vi "Dashboard Main.vi"() -> ()   [LabVIEW 2014]
uses:
  <vilib>/event_ctls.llb/eventvkey.ctl
  <vilib>/Rock Robotics/WPI/Dashboard/WPI_DashboardLogging Global.vi
  <vilib>/Rock Robotics/Network Tables/SD Write Numeric Array.vi
  <vilib>/Rock Robotics/Network Tables/SD Write Number.vi
  <vilib>/Rock Robotics/Network Tables/SD Write String Array.vi
  <vilib>/Rock Robotics/Network Tables/SD Read String Array.vi
  <vilib>/Rock Robotics/Network Tables/SD Write Boolean.vi
  <vilib>/Utility/config.llb/Write Key (String).vi
  <vilib>/Utility/config.llb/Write Key (I32).vi
  <vilib>/Utility/config.llb/NI_LVConfig.lvlib
panel:
  in  "Close Dashboard":bool
  in  "TCP":refnum<k5>
  in  "Rec Mode":enum32{"Stop", "Record", "Playback"}(radio)
  in  "Vision":u16(ring) items=["Camera Off", "USB Camera SW", "USB Camera HW", "IP Camera"]
  out "Camera IP":string
  out "Image Message":string="Timeout in Camera Communications"
  in  "Dashboard Tab":T1(tab)
  in  "Camera Settings":T2={"Frame Rate"=30, "Compression"=30, "Size"=1} {"Frame Rate" scale=1.0..30.0; "Size" items=["640x480", "320x240", "160x120"]}
  out "MotorChart R":cluster{"Numeric":dbl, "Numeric":dbl}(graph)
  out "MotorChart L":T3(graph)
  out "MotorSliders R":cluster{"MotorSlide1":dbl, "MotorSlide2":dbl} {"MotorSlide2" scale=-1.0..1.0 scale format="%#_2e"; "MotorSlide1" scale=-1.0..1.0 scale format="%#_2e"}
  out "MotorSliders L":T4 {"MotorSlide4 2" scale=0.0..14.0 scale format="%#_2e"; "MotorSlide2" scale=-1.0..1.0 scale format="%#_2e"; "MotorSlide1" scale=-1.0..1.0 scale format="%#_2e"}
  out "JS1 Z":dbl(slide) scale=-1.0..1.0 scale format="%#_2e"
  out "JS1 Graph":cluster{"X":dbl, "Y":dbl}[](graph)
  out "JS1 Buttons":T5
  out "JS2 Z":dbl(slide) scale=-1.0..1.0 scale format="%#_2e"
  out "JS2 Graph":cluster{"X":dbl, "Y":dbl}[](graph)
  out "JS2 Buttons":T5
  out "Mode":T6(ring)=enum."Auto Disabled"
  in  "DB Camera Config":bool
  out "fps":dbl format="%#.1g"
  out "Mbps":dbl format="%#.1g"
  out "Mbps 2":bool
  out "Compass":dbl(knob)
  in  "DB/String 9":string
  in  "DB/String 8":string
  in  "DB/String 7":string
  in  "DB/String 6":string
  in  "DB/String 5":string
  in  "DB/String 4":string
  in  "DB/String 3":string
  in  "DB/String 2":string
  in  "DB/String 1":string
  in  "DB/String 0":string
  in  "DB/Slider 0":dbl(slide) scale=0.0..5.0
  in  "DB/Slider 1":dbl(slide) scale=0.0..5.0
  in  "DB/Slider 2":dbl(slide) scale=0.0..5.0
  in  "DB/Slider 3":dbl(slide) scale=0.0..5.0
  out "DB/LED 3":bool
  out "DB/LED 2":bool
  out "DB/LED 1":bool
  out "DB/LED 0":bool
  in  "DB/Button 3":bool
  in  "DB/Button 2":bool
  in  "DB/Button 1":bool
  in  "DB/Button 0":bool caption="New Name"
  in  "Clear Faults Joysticks":T7(ring)=enum."7 Left"
  in  "Toggle Field Centric \nJoysticks":T7(ring)=enum."3 Right"
  in  "Drive Reduction Joysticks":T7(ring)
  in  "Gyro Reset Joysticks":T7(ring)=enum."3 Left"
  in  "Toggle Field Centric\nXbox":T8(ring)=enum."Left bumper"
  in  "Gyro reset Xbox":T8(ring)=enum."Left bumper"
  in  "Drive reduction Xbox":T8(ring)=enum."Left bumper"
  in  "Clear Faults Xbox":T8(ring)=enum."Left bumper"
  in  "Rotate Joysticks":T9(ring)=enum."X right"
  in  "Translate Y Joysticks":T9(ring)=enum."Y left"
  in  "Translate X Joysticks":T9(ring)
  in  "Rotate Xbox":T10(ring)=enum."Right X"
  in  "Translate Y Xbox":T10(ring)
  in  "Translate X Xbox":T10(ring)=enum."Left Y"
  in  "Primary Mode":enum16{"Joysticks", "Xbox"}(ring)
  in  "Low elevator":T8(ring)=enum."Left bumper"
  in  "Axis for manual Control of \narm":T10(ring)
  in  "High elevator":T8(ring)=enum."Right bumper"
  in  "Claw up":T8(ring)
  in  "Claw Down":T8(ring)=enum."B"
  in  "Axis for manual Control of Claw":T10(ring)=enum."Right X"
  in  "Rotate Claw":T10(ring)=enum."Right trigger"
  in  "Open/Close claw":T8(ring)=enum."Y"
  in  "Enable Manual Claw":T8(ring)=enum."Right bumper"
  in  "Enable Manual Elevator":T8(ring)=enum."Right bumper"
  in  "Lift":T8(ring)=enum."Right bumper"
  in  "Middle Lift":T8(ring)=enum."Right bumper"
  in  "Middle Claw":T8(ring)=enum."Right bumper"
  in  "Test Slider":dbl(slide) scale=0.0..100.0 scale format="%#_3g"
  in  "On/Off":bool caption="Solenoid"
  in  "Test Name":u16(ring) items=["Select the test to run...", "Example Test", "-------------------------------", "List of tests is built in robot code.", "Replace with your own automated tests."]
  in  "Test Tree":string(tree)
  in  "Motor":cluster{"Value":dbl, "Enable":bool} {"Value" scale=-1.0..1.0 scale format="%#_3g"}
  out "Progress":T11 {"Test Progress" scale=0.0..100.0}
  in  "Rev/Fwd":cluster{"Forward":bool, "Reverse":bool}
  in  "Test Ring":u16(ring) items=["Monochrome", "Color"]
  in  "Listbox":i32(listbox)
  out "Tree":string(tree)
  in  "?":bool
  in  "Variables":string[](array[string])
  out "Camera Image":T12(plugin-control)
  out "Boolean":bool
  # "Left"
  # "Front"
  # "Right"
  # "Battery"
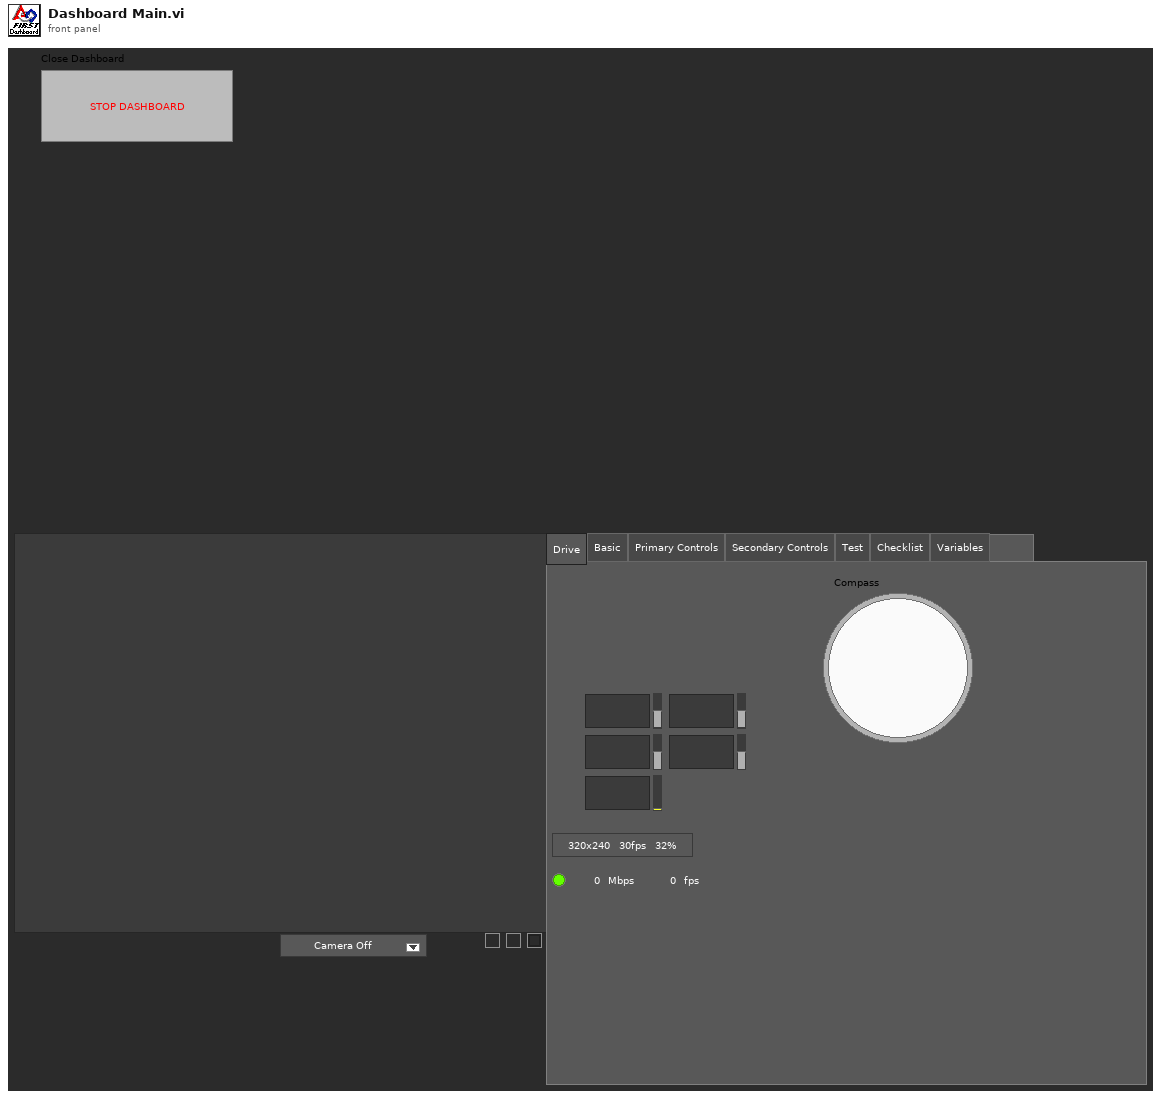
[diagram p1: front panel]
types:
  T1 = enum32{"Drive", "Basic", "Primary Controls", "Secondary Controls", "Test", "Checklist", "Variables"}
  T2 = cluster{"Frame Rate":i32, "Compression":i32, "Size":u16}
  T3 = cluster{"Numeric":dbl, "Numeric":dbl, "Battery V":dbl}
  T4 = cluster{"MotorSlide1":dbl, "MotorSlide2":dbl, "MotorSlide4 2":dbl}
  T5 = cluster{bool, bool, bool, bool, bool, bool, bool, bool, bool, bool, bool, bool}
  T6 = enum8{"Tele-Op Disabled", "Tele-Op Enabled", "Auto Disabled", "Auto Enabled", "Test Disabled", "Test Enabled", "Disconnected", "No Code", "E-Stop"}
  T7 = enum16{"Trigger Left", "2 Left", "3 Left", "4 Left", "5 Left", "6 Left", "7 Left", "8 Left", "9 Left", "10 Left", "11 Left", "Trigger Right", "2 Right", "3 Right", "4 Right", "5 Right", "6 Right", "7 Right", "8 Right", "9 Right", "10 Right", "11 Right"}
  T8 = enum16{"A", "B", "X", "Y", "Left bumper", "Right bumper", "Back", "Start", "Left Joystick down", "Right Joystick down"}
  T9 = enum16{"X left ", "Y left", "Z left", "X right", "Y right", "Z right"}
  T10 = enum16{"Left X", "Left Y", "Left trigger", "Right trigger", "Right X", "Right Y"}
  T11 = cluster{"Test Progress":u8, "Test Progress Text":string}
  T12 = typedef "IMAQ Image.ctl" = refnum<image>
  T13 = enum32{"Drive", "Basic", "Custom", "Test", "Checklist", "Variables"}
  T14 = typedef "Image Type" = u32
  T15 = enum16{"X left ", "Y left", "Z left", "X right", "Y right", "Z right"}[]
  T16 = enum16{"Trigger Left", "2 Left", "3 Left", "4 Left", "5 Left", "6 Left", "7 Left", "8 Left", "9 Left", "10 Left", "11 Left", "Trigger Right", "2 Right", "3 Right", "4 Right", "5 Right", "6 Right", "7 Right", "8 Right", "9 Right", "10 Right", "11 Right"}[]
  T17 = enum16{"Left X", "Left Y", "Left trigger", "Right trigger", "Right X", "Right Y"}[]
  T18 = enum16{"A", "B", "X", "Y", "Left bumper", "Right bumper", "Back", "Start", "Left Joystick down", "Right Joystick down"}[]
  T19 = cluster{"Error Strings":string, "Disable Counts":cluster{u16, u16}, "Rail Faults":cluster{u16, u16, u16}, "Robot IP":string, "DB Mode":u8, "Event Info":cluster{"Name":string, "Type":u8, "Number":u16, "Replay":u8}, "Camera Addr":string}
  T20 = cluster{"Storage":cluster{"Disk Free":u64, "RAM Block":u32, "RAM free":u32}, "CPU Utilization":cluster{"CPU % ISR":sgl, "CPU % Time Crit":sgl, "CPU % Timed Str":sgl, "CPU % High":sgl, "CPU % Above":sgl, "CPU % Normal":sgl, "CPU % Low":sgl}, "CAN":cluster{"% Bus Utilization":sgl, "Bus Off Cnt":u32, "TX_FIFO Full Cnt":u32, "Receive Error Cnt":u8, "Transmit Error Cnt":u8}, "HID":cluster{"HID Outputs":u32, "Rumble Low":u16, "Rumble High":u16}[]}
  T21 = cluster{"Status bits":cluster{"Test Mode":bool, "Autonomous":bool, "Enabled":bool, "Code Start":bool, "Brownout":bool, "Reserved 2":bool, "Reserved 3":bool, "E-Stop":bool}, "Code Trace":cluster{"Disabled":bool, "TeleOp":bool, "Auto":bool, "Test":bool}, "Controller Type":enum16{"unknown", "cRIO", "roboRio"}, "Code?":enum16{"unknown", "noCode", "code"}, "Battery V":dbl}
  T22 = cluster{"Control Bits":cluster{"TestMode":bool, "Autonomous":bool, "Enabled":bool, "FMS Present":bool, bool, bool, bool, "E-Stop":bool}, "Team Station ":u8, "Countdown":sgl, "Joystick Values":cluster{"Axes":dbl[], "Buttons":bool[], "POVs":i16[]}[]}
  T23 = cluster{"Axes":dbl[], "Buttons":bool[], "POVs":i16[]}[]
  T24 = cluster{"Axes":dbl[], "Buttons":bool[], "POVs":i16[]}
  T25 = cluster{"Buttons[0]":bool, "Buttons[1]":bool, "Buttons[2]":bool, "Buttons[3]":bool, "Buttons[4]":bool, "Buttons[5]":bool, "Buttons[6]":bool, "Buttons[7]":bool, "Buttons[8]":bool, "Buttons[9]":bool, "Buttons[10]":bool, "Buttons[11]":bool}
  T26 = cluster{"Camera Image":refnum<vi>, "Dashboard Tab":refnum<vi>, "Boolean":refnum<vi>, "Vision":refnum<vi>, "Rec Mode":refnum<vi>, "Test Slider":refnum<vi>, "On/Off ":refnum<vi>, "Test Ring":refnum<vi>, "Rev/Fwd":refnum<vi>, "Test Name":refnum<vi>, "Motor":refnum<vi>, "Progress":refnum<vi>, "CheckList":refnum<vi>, "Tree":refnum<vi>, "Test Tree":refnum<vi>}
  T27 = typedef "NI_LVConfig.lvlib/Config Data RefNum.ctl" = refnum<k1>
  T28 = cluster{"Operation":enum16{"Update", "Clear"}, "Color Box":u32}[]
  T29 = typedef "eventvkey.ctl" = enum16{"ASCII", "Enter", "Return", "Shift", "Ctrl", "Alt", "Cmd", "Opt", "Caps", "NumLock", "Clear", "Break", "Up", "Down", "Left", "Right", "Insert", "Delete", "Home", "End", "PageUp", "PageDown", "Escape", "Help", "Pause", "ScrollLock", "F1", "F2", "F3", "F4", "F5", "F6", "F7", "F8", "F9", "F10", "F11", "F12", "F13", "F14", "F15", "F16", "F17", "F18", "F19", "F20", "F21", "F22", "F23", "F24", "Play", "VolumeUp", "VolumeDown", "Mute", "Two Byte Char"}
  T30 = cluster{"Image Size":bool, "Image Type":bool, "Pixel Value":bool, "ROI Information":bool, "Zoom Factor":bool}
  T31 = enum8{"Enabled", "Disabled", "Disabled and Grayed Out"}
  T32 = cluster{"Operation":enum16{"Update", "Clear"}, "Color Box":u32}
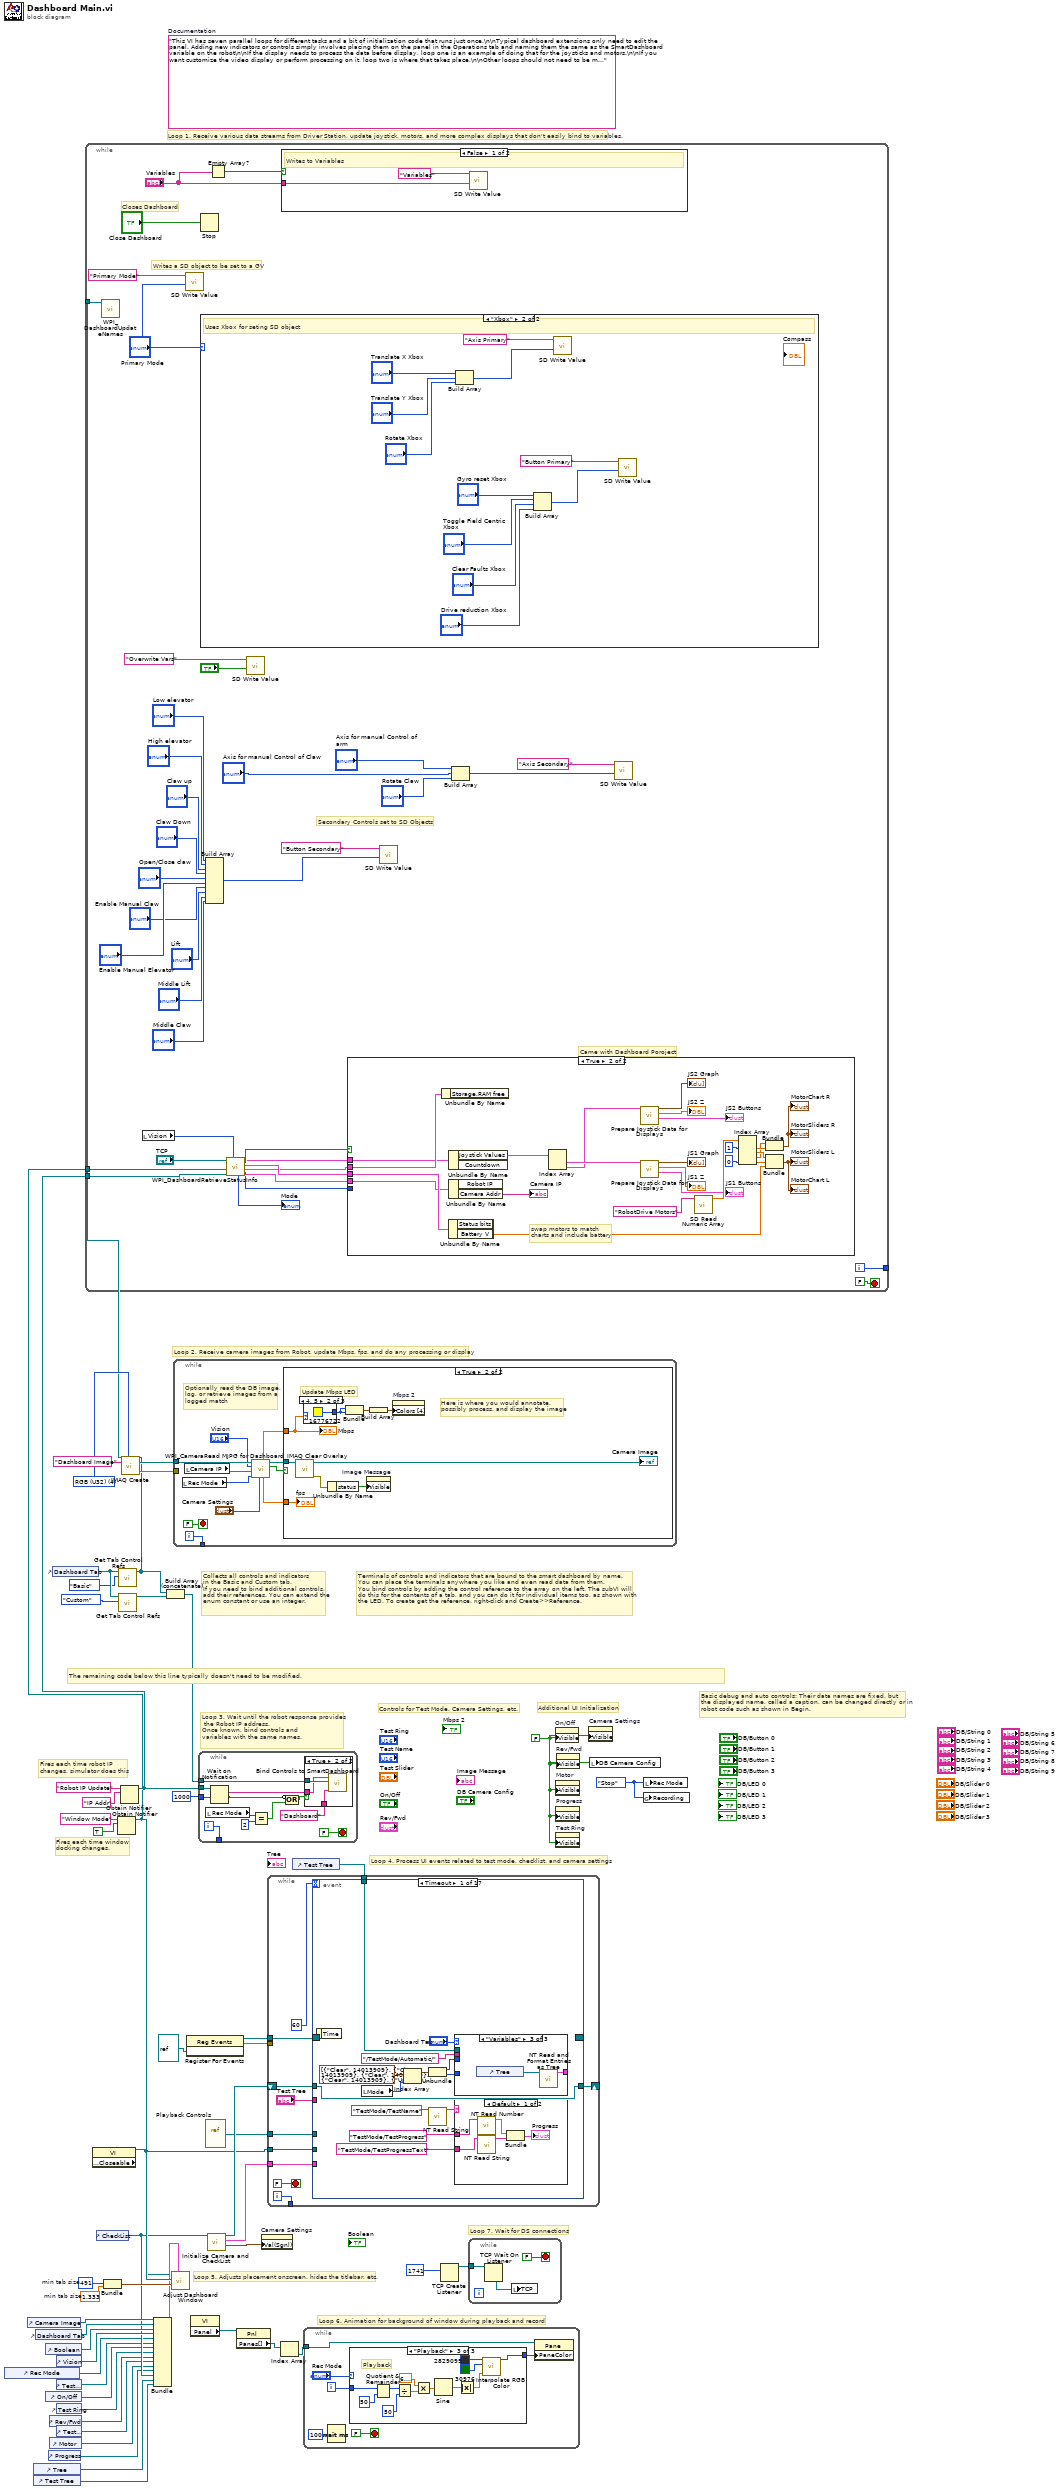
[diagram p0: block diagram]
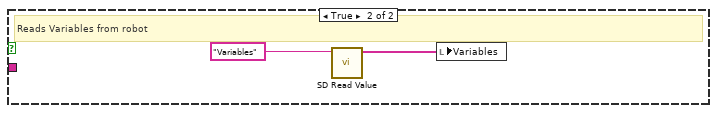
[diagram p2: hidden frame]
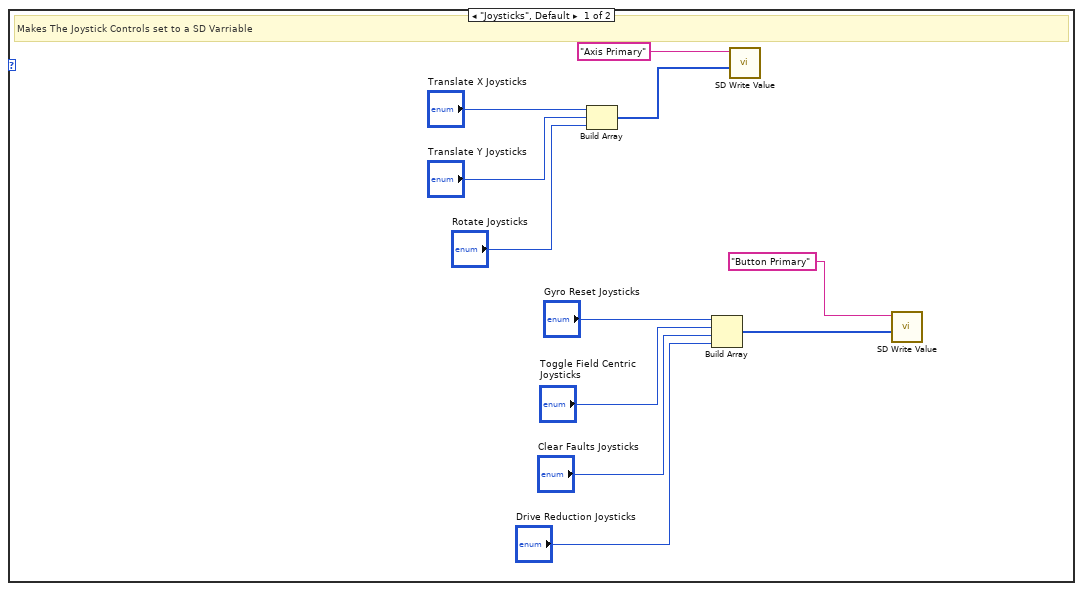
[diagram p3: hidden frame]
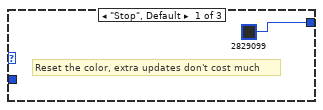
[diagram p5: hidden frame]
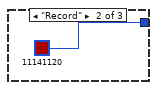
[diagram p6: hidden frame]
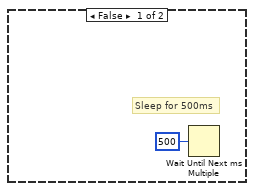
[diagram p8: hidden frame]
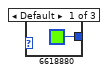
[diagram p9: hidden frame]
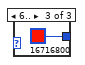
[diagram p10: hidden frame]
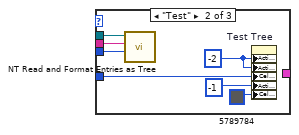
[diagram p12: hidden frame]
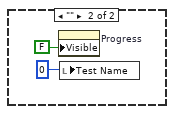
[diagram p13: hidden frame]
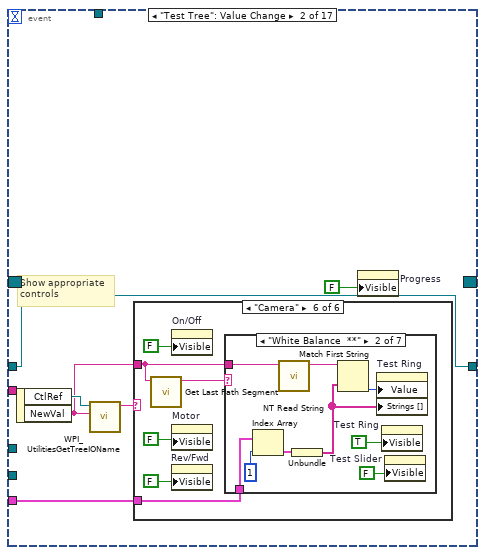
[diagram p14: hidden frame]
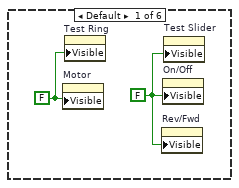
[diagram p15: hidden frame]
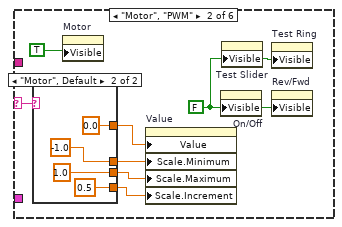
[diagram p16: hidden frame]
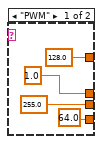
[diagram p17: hidden frame]
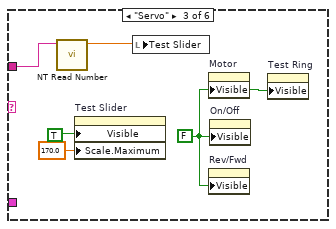
[diagram p18: hidden frame]
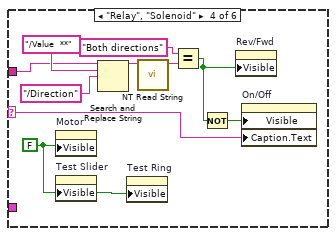
[diagram p19: hidden frame]
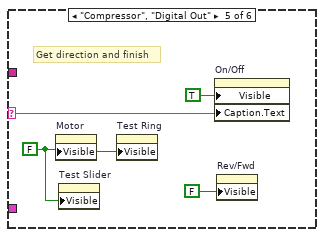
[diagram p20: hidden frame]
diagram:
  w24 = 491  # min tab size
  w23 = 1.333  # min tab size
  w32 = enum32{"Stop", "Record", "Playback"}."Stop" ("Rec Mode")
  w6 = FALSE ("Visible")
  (unwired) "This VI has seven parallel loops for different tasks and a bit of initialization code that runs just once.\n\nTypical dashboard extensions only need to edit the panel. Adding new indicators or controls simply involves placing them on the panel in the Operations tab and naming them the same as the SmartDashboard variable on the robot\n\nIf the display needs to process the data before display, loop one is an example of doing that for the joysticks and motors.\n\nIf you want customize the video display or perform processing on it, loop two is where that takes place.\n\nOther loops should not need to be modified. They are pretty standard, and document the task they perform."  # Documentation
  w52 = T14 4 items=["Grayscale (U8)", "Grayscale (I16)", "Grayscale (SGL)", "Complex (CSG)", "RGB (U32)", "HSL (U32)", "RGB (U64)"] ("Image Type")
  # "Loop 7. Wait for DS connections"
  # "Basic debug and auto controls: Their data names are fixed, but\nthe displayed name, called a caption, can be changed directly or in\nrobot code such as shown in Begin."
  # "Controls for Test Mode, Camera Settings, etc."
  # "Additional UI Initialization"
  # "Loop 6. Animation for background of window during playback and record"
  # "Fires each time robot IP\nchanges, simulator does this"
  # "Fires each time window\ndocking changes."
  # "Collects all controls and indicators\nin the Basic and Custom tab.\nIf you need to bind additional controls,\nadd their references. You can extend the\nenum constant or use an integer."
  # "The remaining code below this line typically doesn't need to be modified."
  # "Loop 4. Process UI events related to test mode, checklist, and camera settings"
  # "Terminals of controls and indicators that are bound to the smart dashboard by name.\nYou can place the terminals anywhere you like and even read data from them.\nYou bind controls by adding the control reference to the array on the left. The subVI will\ndo this for the contents of a tab, and you can do it for individual items too, as shown with\nthe LED. To create get the reference, right-click and Create>>Reference."
  # "Loop 3. Wait until the robot response provides\n the Robot IP address.\nOnce known, bind controls and\nvariables with the same names."
  # "Loop 5. Adjusts placement onscreen, hides the titlebar, etc."
  # "Loop 1. Receive various data streams from Driver Station, update joystick, motors, and more complex displays that don't easily bind to variables."
  # "Loop 2. Receive camera images from Robot, update Mbps, fps, and do any processing or display"
  n1 = control-ref of="Rec Mode"() -> (w12:refnum<vi>)
  n2 = control-ref of="Camera Image"() -> (w27:refnum<vi>)
  n3 = control-ref of="Tree"() -> (w16:refnum<vi>)
  n4 = control-ref of="Test Tree"() -> (w15:refnum<vi>)
  n5 = control-ref of="Dashboard Tab"() -> (w26:refnum<vi>)
  n6 = control-ref of="Boolean"() -> (w21:refnum<vi>)
  n7 = control-ref of="On/Off"() -> (w10:refnum<vi>)
  n8 = control-ref of="Progress"() -> (w7:refnum<vi>)
  n9 = control-ref of="Rev/Fwd"() -> (w8:refnum<vi>)
  n10 = control-ref of="Motor"() -> (w13:refnum<vi>)
  n11 = control-ref of="Dashboard Tab"() -> (w30:refnum<vi>)
  n12 = control-ref of="Test Slider"() -> (w11:refnum<vi>)
  n13 = control-ref of="Vision"() -> (w25:refnum<vi>)
  n14 = control-ref of="Test Ring"() -> (w9:refnum<vi>)
  n15 = control-ref of="Test Name"() -> (w14:refnum<vi>)
  n16 = property class="VI" props=["Front Panel.Closeable"]() -> (reference out=w31:refnum<vi>)  [unwired: 2 in, 2 out]
  n17 = control-ref of="CheckList"() -> (w17:refnum<vi>)
  n18 = Bundle("min tab size"=w24, "min tab size"=w23) -> (w22:cluster{"min tab size":i32, "min tab size":dbl})  [unwired: 1 in]
  n19 = Obtain Notifier(name (unnamed)="Window Mode", notification data type=TRUE) -> (notifier out=w3:refnum<notifier>)  [unwired: 2 in, 2 out]
  n20 = call <vilib>:"Get Tab Control Refs.vi"("Page Index"=T13."Basic" ("Dashboard Tab"), "TabControl in"=w30) -> ("ControlsOnPage"=w4:refnum<vi>[])  [unwired: 9 in]
  n21 = call <vilib>:"Get Tab Control Refs.vi"("Page Index"=T13."Custom" ("Dashboard Tab"), "TabControl in"=w30) -> ("ControlsOnPage"=w29:refnum<vi>[])  [unwired: 9 in]
  n22 = Obtain Notifier(name (unnamed)="Robot IP Update", notification data type="IP Addr" ("name (unnamed)")) -> (notifier out=w5:refnum<notifier>)  [unwired: 2 in, 2 out]
  n23 = while {
    tunnel: [w88] -> _
    tunnel: w5 -> [w82]
    tunnel: w4 -> [w81]
    tunnel: w3 -> [w77]
    i -> [w88]
    stop <- FALSE stop-if-true
    # "Closes Dashboard"
    # "Came with Dashboard Poroject"
    # "Writes a SD object to be set to a GV"
    # "Secondary Controls set to SD Objects"
    n24 = call <vilib>:"WPI_DashboardUpdateNames.vi"("Controls on Tab"=w81) -> ()  [unwired: 11 in]
    n25 = local read "Vision"() -> (w79:u16)
    n26 = call-poly <vilib>:"SD Write Value.vi"("Numeric"="Primary Mode", "Name"="Primary Mode") -> ()  [unwired: 8 in, 2 out]
    n27 = Stop(stop? (T)="Close Dashboard") -> ()
    n28 = case shown="\"Xbox\"" "Primary Mode" {
      frame "Joysticks", Default {
        # "Makes The Joystick Controls set to a SD Varriable"
        n29 = Build Array("Translate X Joysticks", "Translate Y Joysticks", "Rotate Joysticks") -> (w104:T15)
        n30 = Build Array("Gyro Reset Joysticks", "Toggle Field Centric \nJoysticks", "Clear Faults Joysticks", "Drive Reduction Joysticks") -> (w97:T16)
        n31 = call-poly <vilib>:"SD Write Value.vi"("Numeric Array"=w104, "Name"="Axis Primary") -> ()  [unwired: 8 in, 2 out]
        n32 = call-poly <vilib>:"SD Write Value.vi"("Numeric Array"=w97, "Name"="Button Primary") -> ()  [unwired: 8 in, 2 out]
      }
      frame "Xbox" {
        # "Uses Xbox for seting SD object"
        n33 = Build Array("Translate X Xbox", "Translate Y Xbox", "Rotate Xbox") -> (w112:T17)
        n34 = Build Array("Gyro reset Xbox", "Toggle Field Centric\nXbox", "Clear Faults Xbox", "Drive reduction Xbox") -> (w115:T18)
        n35 = call-poly <vilib>:"SD Write Value.vi"("Numeric Array"=w112, "Name"="Axis Primary") -> ()  [unwired: 8 in, 2 out]
        n36 = call-poly <vilib>:"SD Write Value.vi"("Numeric Array"=w115, "Name"="Button Primary") -> ()  [unwired: 8 in, 2 out]
      }
    }
    n37 = Build Array("Low elevator", "High elevator", "Claw up", "Claw Down", "Open/Close claw", "Enable Manual Elevator", "Enable Manual Claw", "Lift", "Middle Lift", "Middle Claw") -> (w75:T18)
    n38 = Empty Array?(array="Variables") -> (empty?=w59:bool)
    n39 = call <vilib>:"WPI_DashboardRetrieveStatusInfo.vi"("Vision"=w79, "Binding Refnum"=w82, "Window Mode Notifier"=w77, "TCP Cnx"="TCP") -> ("Power and Errors"=w83:T19, "Robot Metrics"=w86:T20, "Status Info"=w87:T21, "Control Info"=w84:T22, "Robot Mode"=w80:T6, "Process?"=w85:bool)  [unwired: 2 in]
    "Mode" <- w80
    n40 = call-poly <vilib>:"SD Write Value.vi"("Boolean"="?", "Name"="Overwrite Vars") -> ()  [unwired: 8 in, 2 out]
    n41 = case shown="False" w59 {
      tunnel: "Variables" -> [w90 _]
      frame False {
        # "Writes to Variables"
        n42 = call-poly <vilib>:"SD Write Value.vi"("String Array"=w90, "Name"="Variables") -> ()  [unwired: 8 in, 2 out]
      }
      frame True {
        # "Reads Variables from robot"
        n43 = call-poly <vilib>:"SD Read Value.vi"("Name"="Variables") -> ("String Array"=w92:string[])  [unwired: 9 in, 1 out]
        n44 = local write "Variables"(w92) -> ()
      }
    }
    n45 = case shown="True" w85 {
      tunnel: w87 -> [_ w140]
      tunnel: w86 -> [_ w139]
      tunnel: w84 -> [_ w138]
      tunnel: w83 -> [_ w137]
      tunnel: w80 -> [_ _]
      frame False {
      }
      frame True {
        # "swap motors to match\ncharts and include battery"
        n46 = Unbundle By Name(w139) -> ()  [unwired: 1 out]
        n47 = Unbundle By Name(w140) -> ("Battery V"=w126:dbl)  [unwired: 1 out]
        n48 = Unbundle By Name(w138) -> ("Joystick Values"=w125:T23)  [unwired: 1 out]
        n49 = Unbundle By Name(w137) -> ("Camera Addr"=→"Camera IP":string)  [unwired: 1 out]
        n50 = Index Array(array=w125) -> (element #1=w124:T24, element #2=w119:T24)  [unwired: 2 in]
        n51 = call "Prepare Joystick Data for Displays.vi"("Joystick Values"=w119) -> ("Buttons"=→"JS2 Buttons":T25, "Z Axis"=→"JS2 Z":dbl, "Cartesian Data"=→"JS2 Graph":cluster{"X axis":dbl, "X axis":dbl}[])  [unwired: 8 in]
        n52 = call "Prepare Joystick Data for Displays.vi"("Joystick Values"=w124) -> ("Buttons"=→"JS1 Buttons":T25, "Z Axis"=→"JS1 Z":dbl, "Cartesian Data"=→"JS1 Graph":cluster{"X axis":dbl, "X axis":dbl}[])  [unwired: 8 in]
        n53 = call <vilib>:"SD Read Numeric Array.vi"("Name"="RobotDrive Motors") -> ("Numeric Array"=w128:dbl[])  [unwired: 8 in, 2 out]
        n54 = Index Array(array=w128, index #1=1, index #4=0) -> (element #1=w132:dbl, element #2=w133:dbl, element #3=w131:dbl, element #4=w136:dbl)  [unwired: 2 in]
        n55 = Bundle("Numeric"=w131, "Numeric"=w132) -> (→"MotorChart R" →"MotorSliders R":cluster{"Numeric":dbl, "Numeric":dbl})  [unwired: 1 in]
        n56 = Bundle("Numeric"=w133, "Numeric"=w136, "Battery V"=w126) -> (→"MotorChart L" →"MotorSliders L":T3)  [unwired: 1 in]
      }
    }
    n57 = call-poly <vilib>:"SD Write Value.vi"("Numeric Array"=w75, "Name"="Button Secondary") -> ()  [unwired: 8 in, 2 out]
    n58 = Build Array("Axis for manual Control of \narm", "Axis for manual Control of Claw", "Rotate Claw") -> (w57:T17)
    n59 = call-poly <vilib>:"SD Write Value.vi"("Numeric Array"=w57, "Name"="Axis Secondary") -> ()  [unwired: 8 in, 2 out]
  }
  n60 = call "IMAQ Create"("Image Name"="Dashboard Image", "Image Type"=w52) -> ("New Image"=w50:T12, "error out"=w49:errorcluster)  [unwired: 2 in, 1 out]
  n61 = Bundle("Camera Image"=w27, "Dashboard Tab"=w26, "Boolean"=w21, "Vision"=w25, "Rec Mode"=w12, "Test Slider"=w11, "On/Off"=w10, "Test Ring"=w9, "Rev/Fwd"=w8, "Test Name"=w14, "Motor"=w13, "Progress"=w7, "CheckList"=w17, "Tree"=w16, "Test Tree"=w15) -> (w18:T26)  [unwired: 1 in]
  n62 = Build Array (concatenate)(w4, w29) -> (w28:refnum<vi>[])
  n63 = call "Adjust Dashboard Window.vi"("Sizing Refnums"=w18, "Size Constraints"=w22, "VI"=w31, "Notifier in"=w3) -> ()  [unwired: 8 in]
  n64 = while {
    tunnel: w50 -> [w149]
    tunnel: w49 -> [_]
    tunnel: [w150] -> _
    i -> [w150]
    stop <- FALSE stop-if-true
    # "Optionally read the DB image,\nlog, or retrieve images from a\nlogged match"
    n65 = local read "Rec Mode"() -> (w143:enum32{"Stop", "Record", "Playback"})
    n66 = local read "Camera IP"() -> (w141:string)
    n67 = call <vilib>:"WPI_CameraRead MJPG for Dashboard.vi"("Camera Settings"="Camera Settings", "Rec Mode"=w143, "Camera IP"=w141, "Camera Mode"="Vision", "Refnum in"=w149) -> ("Active"=w147:bool, "Refnum out"=w148:T12, "FPS"=w146:dbl, "Bandwidth (Mbps)"=w145:dbl)  [unwired: 3 in]
    n68 = case shown="True" w147 {
      tunnel: w148 -> [_ w156]
      tunnel: w145 -> [_ w155]
      tunnel: w146 -> [_ w153]
      frame False {
        # "Sleep for 500ms"
        n69 = Wait Until Next ms Multiple(millisecond multiple=u32 500) -> ()  [unwired: 1 out]
      }
      frame True {
        # "Here is where you would annotate,\npossibly process, and display the image"
        # "Update Mbps LED"
        n70 = call "IMAQ Clear Overlay"("Image"=w156) -> ("error out"=w160:errorcluster, "Image Out"=→"Camera Image":T12)  [unwired: 2 in, 7 out]
        n71 = case shown="4, 5" w155 {
          tunnel: [u32 6618880 ("Color Box") u32 16776722 ("Color Box") u32 16716800 ("Color Box")] -> w157
          frame Default {
          }
          frame 4, 5 {
          }
          frame 6.. {
          }
        }
        n72 = Unbundle By Name(w160) -> ("status"=w161:bool)
        n73 = Bundle("Color Box"=w157, "Color Box"=w157) -> (w159:cluster{"Color Box":u32, "Color Box":u32})  [unwired: 1 out]
        n74 = property on="Image Message" class="Str"("Visible"=w161) -> ()  [unwired: 2 in, 2 out]
        n75 = Build Array(w159) -> (w158:cluster{"Color Box":u32, "Color Box":u32}[])
        n76 = property on="Mbps 2" class="Bool (strict)"("Colors [4]"=w158) -> ()  [unwired: 2 in, 2 out]
        "Mbps" <- w155
        "fps" <- w153
      }
    }
  }
  n77 = register-events(refnum<vi> refnum) -> (reference out=w36:refnum<event-registration>, error out=w35:errorcluster)  [unwired: 2 in]
  n78 = property class="VI"() -> ("Panel"=w39:refnum<vi>)  [unwired: 2 in, 2 out]
  n79 = while {
    tunnel: w28 -> [w176]
    tunnel: w5 -> [w174]
    tunnel: [w172] -> _
    tunnel: u32 1000 ("milliseconds to wait") -> [w171]
    i -> [w172]
    stop <- FALSE stop-if-true
    n80 = local read "Rec Mode"() -> (w167:enum32{"Stop", "Record", "Playback"})
    n81 = Wait on Notification(notifier=w174, timeout in ms (-1)=w171) -> (notification=w173:string, timed out?=w169:bool)  [unwired: 2 in, 2 out]
    n82 = Equal?(x=w167, y=u16 2 ("Rec Mode")) -> (x = y?=w168:bool)
    n83 = Compound Arithmetic op=OR(invert w169, w168) -> (w170:bool)
    n84 = case shown="True" w170 {
      tunnel: w176 -> [_ w179]
      tunnel: w173 -> [_ w178]
      tunnel: "Dashboard" -> [_ w177]
      frame False {
      }
      frame True {
        n85 = call <vilib>:"Bind Controls to SmartDashboard.vi"("Client Name"=w177, "Bound Control Refs"=w179, "Server IP Address"=w178) -> ()  [unwired: 9 in]
      }
    }
  }
  n86 = vi-ref "Playback Controls.vi"() -> (w37:refnum<vi>)
  n87 = call "Initialize Camera and CheckList.vi"("ListBox in"=w17) -> ("Cluster"=w43:cluster{"value":i32, "value":i32, "index":i32}, "Array"=w44:cluster{string[]}[], "File Refnum"=w42:T27)  [unwired: 8 in]
  n88 = property class="Pnl"(reference=w39) -> ("Panes[]"=w40:refnum<vi>[])  [unwired: 1 in, 2 out]
  n89 = property on="Camera Settings" class="Clust (strict)"("Val(Sgnl)"=w43) -> ()  [unwired: 2 in, 2 out]
  n90 = Index Array(array=w40) -> (element=w38:refnum<vi>)  [unwired: 1 in]
  n91 = control-ref of="Test Tree"() -> (w41:refnum<vi>)
  n92 = while {
    tunnel: w44 -> [w187]
    shift-right: [w186] -> _
    shift-left: w42 -> [w185]
    tunnel: [w184] -> _
    tunnel: w41 -> [w183]
    tunnel: w37 -> [w182]
    tunnel: w36 -> [w181]
    tunnel: w35 -> [_]
    tunnel: w31 -> [w180]
    i -> [w184]
    stop <- FALSE stop-if-true
    n93 = event shown="[0] Timeout" {
      selector: w181 -> [_ _ _ _ _ _ _ _ _ _ _ _ _ _ _ _ _]
      dyn-events: [_ _ _ _ _ _ _ _ _ _ _ _ _ w425 _ _ _] -> _
      timeout: u32 60 ("milliseconds to wait") -> [_ _ _ _ _ _ _ _ _ _ _ _ _ _ _ _ _]
      tunnel: w183 -> [w199 _ _ _ _ _ _ _ _ _ _ _ _ _ _ _ _]
      tunnel: "Test Tree" -> [_ _ _ _ _ _ _ _ w394 w402 w404 w408 w416 _ _ _ _]
      tunnel: w187 -> [_ w221 _ _ _ _ w358 w388 _ _ _ _ _ _ _ _ _]
      tunnel: [w195 w220 w319 w324 w332 w344 w357 w381 w393 w400 w403 w407 w415 w427 w441 w442 w452] -> w186
      tunnel: w185 -> [w195 w220 w319 w324 w332 w344 w356 w381 w393 w400 w403 w407 w415 w427 w441 w442 w452]
      tunnel: w182 -> [_ _ _ _ _ _ _ _ _ _ _ _ _ w428 _ w445 _]
      tunnel: w180 -> [_ _ _ _ _ _ _ _ _ _ _ _ _ w423 _ _ _]
      event Timeout {
        n94 = event-data() -> ()  [unwired: 1 in, 1 out]
        n95 = local read "Mode"() -> (w198:T6)
        n96 = Index Array(array=T28 [{"Operation"=enum."Clear", "Color Box"=14013909}, {"Operation"=enum."Clear", "Color Box"=14013909}, {"Operation"=enum."Clear", "Color Box"=14013909}, {"Operation"=enum."Clear", "Color Box"=14013909}, {"Operation"=enum."Update", "Color Box"=14013909}, {"Operation"=enum."Update", "Color Box"=16777215}, {"Operation"=enum."Clear", "Color Box"=14013909}, {"Operation"=enum."Clear", "Color Box"=14013909}, {"Operation"=enum."Clear", "Color Box"=14013909}], index=w198) -> (element=w193:T32)
        n97 = Unbundle(w193) -> ("Operation"=w192:enum16{"Update", "Clear"}, "Color Box"=w191:u32)
        n98 = call <vilib>:"NT Read String.vi"("Name"="TestMode/TestName") -> ("String"=w202:string)  [unwired: 9 in, 1 out]
        n99 = case shown="\"Variables\"" "Dashboard Tab" {
          tunnel: w199 -> [_ w210 _]
          tunnel: "/TestMode/Automatic/" ("Name Pattern") -> [_ w209 _]
          tunnel: w192 -> [_ w208 _]
          tunnel: [_ _ w212] -> _
          tunnel: w191 -> [_ w204 _]
          frame "Primary Controls", Default {
          }
          frame "Test" {
            w207 = -2 ("Active Item:Row Number")
            n100 = call <vilib>:"NT Read and Format Entries as Tree.vi"("Operation"=w208, "Name Pattern"=w209, "Tree Refnum"=w210) -> ()  [unwired: 7 in, 2 out]
            n101 = property on="Test Tree" class="Tree (strict)"("Active Item Row Number"=w207, "ActiveColNum"=w207, "CellBG"=w204, "Active Item Row Number"=-1 ("Active Item:Row Number"), "CellBG"=u32 5789784 ("Color Box")) -> ()  [unwired: 2 in, 2 out]
          }
          frame "Variables" {
            n102 = control-ref of="Tree"() -> (w211:refnum<vi>)
            n103 = call <vilib>:"NT Read and Format Entries as Tree.vi"("Tree Refnum"=w211) -> ("Formatted Strings"=w212:cluster{"Name":string, "Value":string}[])  [unwired: 9 in, 1 out]
          }
        }
        n104 = case shown="Default" w202 {
          tunnel: "TestMode/TestProgress" ("Name") -> [w214 _]
          tunnel: "TestMode/TestProgressText" ("Name") -> [w213 _]
          frame Default {
            n105 = call <vilib>:"NT Read Number.vi"("Name"=w214) -> ("Numeric"=w215:dbl)  [unwired: 9 in, 1 out]
            n106 = call <vilib>:"NT Read String.vi"("Name"=w213) -> ("String"=w216:string)  [unwired: 9 in, 1 out]
            n107 = Bundle("Numeric"=w215, "String"=w216) -> (→"Progress":cluster{"Numeric":dbl, "String":string})  [unwired: 1 in]
          }
          frame "" {
            n108 = property on="Progress" class="Clust (strict)"("Visible"=FALSE) -> ()  [unwired: 2 in, 2 out]
            n109 = local write "Test Name"(u16 0) -> ()
          }
        }
      }
      event "Test Tree": Value Change {
        # "Show appropriate\ncontrols"
        n110 = event-data() -> ("CtlRef"=w224:refnum<vi>, "NewVal"=w222:string)  [unwired: 1 in]
        n111 = call <vilib>:"WPI_UtilitiesGetTreeIOName.vi"("NewVal"=w222, "TreeControl in"=w224) -> ("I/O Name"=w225:string)  [unwired: 9 in]
        n112 = case shown="\"Camera\"" w225 {
          selector: w225 -> [_ w232 _ w250 w259 _]
          tunnel: w222 -> [_ _ w247 w249 _ w266]
          tunnel: w221 -> [_ _ _ _ _ w265]
          frame Default {
            w227 = FALSE ("Visible")
            w226 = FALSE ("Visible")
            n113 = property on="Motor" class="Clust (strict)"("Visible"=w226) -> ()  [unwired: 2 in, 2 out]
            n114 = property on="Test Ring" class="Ring (strict)"("Visible"=w226) -> ()  [unwired: 2 in, 2 out]
            n115 = property on="Rev/Fwd" class="Clust (strict)"("Visible"=w227) -> ()  [unwired: 2 in, 2 out]
            n116 = property on="On/Off" class="Bool (strict)"("Visible"=w227) -> ()  [unwired: 2 in, 2 out]
            n117 = property on="Test Slider" class="Slide (strict)"("Visible"=w227) -> ()  [unwired: 2 in, 2 out]
          }
          frame "Motor", "PWM" {
            w233 = FALSE ("Visible")
            n118 = case shown="\"Motor\", Default" w232 {
              tunnel: [1.0 ("Value") -1.0 ("Value")] -> w231
              tunnel: [255.0 ("Value") 1.0 ("Value")] -> w230
              tunnel: [128.0 ("Value") 0.0 ("Value")] -> w229
              tunnel: [64.0 ("Value") 0.5 ("Value")] -> w228
              frame "PWM" {
              }
              frame "Motor", Default {
              }
            }
            n119 = property on="Motor" class="Clust (strict)"("Visible"=TRUE) -> ()  [unwired: 2 in, 2 out]
            n120 = property on="Value" class="Slide (strict)"("Value"=w229, "Scale.Minimum"=w231, "Scale.Maximum"=w230, "Scale.Increment"=w228) -> ()  [unwired: 2 in, 2 out]
            n121 = property on="On/Off" class="Bool (strict)"("Visible"=w233) -> ()  [unwired: 2 in, 2 out]
            n122 = property on="Test Slider" class="Slide (strict)"("Visible"=w233) -> ()  [unwired: 2 in, 2 out]
            n123 = property on="Test Ring" class="Ring (strict)"("Visible"=w233) -> ()  [unwired: 2 in, 2 out]
            n124 = property on="Rev/Fwd" class="Clust (strict)"("Visible"=w233) -> ()  [unwired: 2 in, 2 out]
          }
          frame "Servo" {
            w245 = FALSE ("Visible")
            n125 = call <vilib>:"NT Read Number.vi"("Name"=w247) -> ("Numeric"=w246:dbl)  [unwired: 9 in, 1 out]
            n126 = property on="Test Slider" class="Slide (strict)"("Visible"=TRUE, "Scale.Maximum"=170.0 ("Scale.Range:Maximum")) -> ()  [unwired: 2 in, 2 out]
            n127 = local write "Test Slider"(w246) -> ()
            n128 = property on="Motor" class="Clust (strict)"("Visible"=w245) -> ()  [unwired: 2 in, 2 out]
            n129 = property on="Rev/Fwd" class="Clust (strict)"("Visible"=w245) -> ()  [unwired: 2 in, 2 out]
            n130 = property on="On/Off" class="Bool (strict)"("Visible"=w245) -> ()  [unwired: 2 in, 2 out]
            n131 = property on="Test Ring" class="Ring (strict)"("Visible"=w245) -> ()  [unwired: 2 in, 2 out]
          }
          frame "Relay", "Solenoid" {
            w248 = FALSE ("Visible")
            n132 = property on="Motor" class="Clust (strict)"("Visible"=w248) -> ()  [unwired: 2 in, 2 out]
            n133 = property on="Test Slider" class="Slide (strict)"("Visible"=w248) -> ()  [unwired: 2 in, 2 out]
            n134 = Search and Replace String(input string=w249, search string="/Value  **", replace string="/Direction") -> (result string=w255:string)  [unwired: 5 in, 3 out]
            n135 = property on="Test Ring" class="Ring (strict)"("Visible"=w248) -> ()  [unwired: 2 in, 2 out]
            n136 = call <vilib>:"NT Read String.vi"("Name"=w255) -> ("String"=w253:string)  [unwired: 9 in, 1 out]
            n137 = Equal?(x="Both directions", y=w253) -> (x = y?=w251:bool)
            n138 = Not(x=w251) -> (.not. x?=w252:bool)
            n139 = property on="Rev/Fwd" class="Clust (strict)"("Visible"=w251) -> ()  [unwired: 2 in, 2 out]
            n140 = property on="On/Off" class="Bool (strict)"("Visible"=w252, "Caption.Text"=w250) -> ()  [unwired: 2 in, 2 out]
          }
          frame "Compressor", "Digital Out" {
            w258 = FALSE ("Visible")
            # "Get direction and finish"
            n141 = property on="Motor" class="Clust (strict)"("Visible"=w258) -> ()  [unwired: 2 in, 2 out]
            n142 = property on="Test Slider" class="Slide (strict)"("Visible"=w258) -> ()  [unwired: 2 in, 2 out]
            n143 = property on="Test Ring" class="Ring (strict)"("Visible"=w258) -> ()  [unwired: 2 in, 2 out]
            n144 = property on="On/Off" class="Bool (strict)"("Visible"=TRUE, "Caption.Text"=w259) -> ()  [unwired: 2 in, 2 out]
            n145 = property on="Rev/Fwd" class="Clust (strict)"("Visible"=FALSE) -> ()  [unwired: 2 in, 2 out]
          }
          frame "Camera" {
            n146 = call <vilib>:"Get Last Path Segment.vi"("String in"=w266) -> ("String out"=w267:string)  [unwired: 10 in]
            n147 = property on="On/Off" class="Bool (strict)"("Visible"=FALSE) -> ()  [unwired: 2 in, 2 out]
            n148 = property on="Motor" class="Clust (strict)"("Visible"=FALSE) -> ()  [unwired: 2 in, 2 out]
            n149 = property on="Rev/Fwd" class="Clust (strict)"("Visible"=FALSE) -> ()  [unwired: 2 in, 2 out]
            n150 = case shown="\"White Balance  **\"" w267 {
              tunnel: w266 -> [w273 w282 w291 w300 w309 _ w315]
              tunnel: w265 -> [w271 w279 w288 w297 w306 _ _]
              frame "Size  **" {
                n151 = Index Array(array=w271) -> (element=w270:cluster{string[]})  [unwired: 1 in]
                n152 = call <vilib>:"NT Read String.vi"("Name"=w273) -> ("String"=w272:string)  [unwired: 9 in, 1 out]
                n153 = Unbundle(w270) -> (w268:string[])
                n154 = Match First String(2:w268, 3:w272) -> (0:w269:i32)  [unwired: 1 out]
                n155 = property on="Test Ring" class="Ring (strict)"("Value"=w269, "Strings []"=w268) -> ()  [unwired: 2 in, 2 out]
                n156 = property on="Test Ring" class="Ring (strict)"("Visible"=TRUE) -> ()  [unwired: 2 in, 2 out]
                n157 = property on="Test Slider" class="Slide (strict)"("Visible"=FALSE) -> ()  [unwired: 2 in, 2 out]
              }
              frame "White Balance  **" {
                n158 = Index Array(array=w279, index=1) -> (element=w280:cluster{string[]})
                n159 = call <vilib>:"NT Read String.vi"("Name"=w282) -> ("String"=w281:string)  [unwired: 9 in, 1 out]
                n160 = Unbundle(w280) -> (w277:string[])
                n161 = Match First String(2:w277, 3:w281) -> (0:w276:i32)  [unwired: 1 out]
                n162 = property on="Test Ring" class="Ring (strict)"("Value"=w276, "Strings []"=w277) -> ()  [unwired: 2 in, 2 out]
                n163 = property on="Test Ring" class="Ring (strict)"("Visible"=TRUE) -> ()  [unwired: 2 in, 2 out]
                n164 = property on="Test Slider" class="Slide (strict)"("Visible"=FALSE) -> ()  [unwired: 2 in, 2 out]
              }
              frame "Exposure  **" {
                n165 = Index Array(array=w288, index=2) -> (element=w289:cluster{string[]})
                n166 = call <vilib>:"NT Read String.vi"("Name"=w291) -> ("String"=w290:string)  [unwired: 9 in, 1 out]
                n167 = Unbundle(w289) -> (w285:string[])
                n168 = Match First String(2:w285, 3:w290) -> (0:w286:i32)  [unwired: 1 out]
                n169 = property on="Test Ring" class="Ring (strict)"("Value"=w286, "Strings []"=w285) -> ()  [unwired: 2 in, 2 out]
                n170 = property on="Test Ring" class="Ring (strict)"("Visible"=TRUE) -> ()  [unwired: 2 in, 2 out]
                n171 = property on="Test Slider" class="Slide (strict)"("Visible"=FALSE) -> ()  [unwired: 2 in, 2 out]
              }
              frame "Exposure Priority  **" {
                n172 = Index Array(array=w297, index=3) -> (element=w298:cluster{string[]})
                n173 = call <vilib>:"NT Read String.vi"("Name"=w300) -> ("String"=w299:string)  [unwired: 9 in, 1 out]
                n174 = Unbundle(w298) -> (w294:string[])
                n175 = Match First String(2:w294, 3:w299) -> (0:w295:i32)  [unwired: 1 out]
                n176 = property on="Test Ring" class="Ring (strict)"("Value"=w295, "Strings []"=w294) -> ()  [unwired: 2 in, 2 out]
                n177 = property on="Test Ring" class="Ring (strict)"("Visible"=TRUE) -> ()  [unwired: 2 in, 2 out]
                n178 = property on="Test Slider" class="Slide (strict)"("Visible"=FALSE) -> ()  [unwired: 2 in, 2 out]
              }
              frame "Color Enable  **" {
                n179 = Index Array(array=w306, index=4) -> (element=w307:cluster{string[]})
                n180 = call <vilib>:"NT Read String.vi"("Name"=w309) -> ("String"=w308:string)  [unwired: 9 in, 1 out]
                n181 = Unbundle(w307) -> (w303:string[])
                n182 = Match First String(2:w303, 3:w308) -> (0:w304:i32)  [unwired: 1 out]
                n183 = property on="Test Ring" class="Ring (strict)"("Value"=w304, "Strings []"=w303) -> ()  [unwired: 2 in, 2 out]
                n184 = property on="Test Ring" class="Ring (strict)"("Visible"=TRUE) -> ()  [unwired: 2 in, 2 out]
                n185 = property on="Test Slider" class="Slide (strict)"("Visible"=FALSE) -> ()  [unwired: 2 in, 2 out]
              }
              frame Default {
                n186 = property on="Test Ring" class="Ring (strict)"("Visible"=FALSE) -> ()  [unwired: 2 in, 2 out]
                n187 = property on="Test Slider" class="Slide (strict)"("Visible"=FALSE) -> ()  [unwired: 2 in, 2 out]
              }
              frame "Brightness  **", "Color Level  **", "Compression  **", "FPS  **", "Sharpness  **" {
                n188 = call <vilib>:"NT Read Number.vi"("Name"=w315) -> ("Numeric"=w314:dbl)  [unwired: 9 in, 1 out]
                n189 = local write "Test Slider"(w314) -> ()
                n190 = property on="Test Slider" class="Slide (strict)"("Visible"=TRUE, "Scale.Maximum"=100.0 ("Scale.Range:Maximum")) -> ()  [unwired: 2 in, 2 out]
                n191 = property on="Test Ring" class="Ring (strict)"("Visible"=FALSE) -> ()  [unwired: 2 in, 2 out]
              }
            }
          }
        }
        n192 = property on="Progress" class="Clust (strict)"("Visible"=FALSE) -> ()  [unwired: 2 in, 2 out]
      }
      event "Test Name": Mouse Enter {
        # "Populate the ring with the list of tests"
        n193 = event-data() -> ()  [unwired: 1 in, 1 out]
        n194 = call <vilib>:"NT Read String Array.vi"("Name"="TestMode/TestList") -> ("String Array"=w323:string[])  [unwired: 9 in, 1 out]
        n195 = Build Array (concatenate)("Select the test to run...", w323) -> (w322:string[])
        n196 = property on="Test Name" class="Ring (strict)"("Strings []"=w322) -> ()  [unwired: 2 in, 2 out]
      }
      event "Test Name": Value Change {
        w325 = FALSE ("Visible")
        # "Tell the robot the test name to run"
        n197 = event-data() -> ("NewVal"=w329:u16)  [unwired: 1 in]
        n198 = property on="Test Name" class="Ring (strict)"() -> ("Strings []"=w330:string[])  [unwired: 2 in, 2 out]
        n199 = local write "Progress"(T11 {"Test Progress"=0, "Test Progress Text"=""} ("Progress")) -> ()
        n200 = Index Array(array=w330, index=w329) -> (element=w328:string)
        n201 = call <vilib>:"NT Write String.vi"("String"=w328, "Name"="TestMode/TestName") -> ()  [unwired: 9 in, 1 out]
        n202 = property on="Progress" class="Clust (strict)"("Visible"=TRUE) -> ()  [unwired: 2 in, 2 out]
        n203 = property on="Motor" class="Clust (strict)"("Visible"=w325) -> ()  [unwired: 2 in, 2 out]
        n204 = property on="Test Slider" class="Slide (strict)"("Visible"=w325) -> ()  [unwired: 2 in, 2 out]
        n205 = property on="On/Off" class="Bool (strict)"("Visible"=w325) -> ()  [unwired: 2 in, 2 out]
        n206 = property on="Rev/Fwd" class="Clust (strict)"("Visible"=w325) -> ()  [unwired: 2 in, 2 out]
        n207 = property on="Test Ring" class="Ring (strict)"("Visible"=w325) -> ()  [unwired: 2 in, 2 out]
      }
      event "Listbox": Double Click {
        # "Shift clears all"
        # "Update symbols on the listbox"
        n208 = event-data() -> ("PlatMods.Shift"=w333:bool, "Row"=w335:i32)  [unwired: 1 in]
        n209 = case shown="True" w333 {
          tunnel: w335 -> [w339 _]
          tunnel: 1 -> [w338 _]
          frame False {
            n210 = property on="Listbox" class="LstBox (strict)"() -> ("Item Symbols"=w337:i32[])  [unwired: 2 in, 2 out]
            n211 = Replace Array Subset(array=w337, new element=w338, index=w339) -> (w336:i32[])
            n212 = property on="Listbox" class="LstBox (strict)"("Item Symbols"=w336) -> ()  [unwired: 2 in, 2 out]
          }
          frame True {
            w340 = 0 ("Top Row")
            n213 = property on="Listbox" class="LstBox (strict)"() -> ("Number of Rows"=w342:u32)  [unwired: 2 in, 2 out]
            n214 = Initialize Array(0, w342) -> (w341:i32[])
            n215 = property on="Listbox" class="LstBox (strict)"("Top Row"=w340, "Value"=w340, "Item Symbols"=w341) -> ()  [unwired: 2 in, 2 out]
          }
        }
      }
      event "Listbox": Key Down {
        # "Update symbols on the listbox\nLeft and right keys check and uncheck"
        n216 = event-data() -> ("VKey"=w346:T29)  [unwired: 1 in]
        n217 = case shown="\"Left\", \"Right\"" w346 {
          selector: w346 -> [w351 _]
          tunnel: eventvkey."Left" ("VKey") -> [w349 _]
          frame "Left", "Right" {
            n218 = Equal?(x=w349, y=w351) -> (x = y?=w350:bool)
            n219 = Select(t=0, s=w350, f=1) -> (s? t:f=w352:i32)
            n220 = property on="Listbox" class="LstBox (strict)"() -> ("Item Symbols"=w355:i32[])  [unwired: 2 in, 2 out]
            n221 = Replace Array Subset(array=w355, new element=w352, index="Listbox") -> (w354:i32[])
            n222 = property on="Listbox" class="LstBox (strict)"("Item Symbols"=w354) -> ()  [unwired: 2 in, 2 out]
          }
          frame Default {
          }
        }
      }
      event "DB Camera Config": Value Change {
        # "Show or hide the cluster of controls, store in ini file"
        n223 = event-data() -> ("NewVal"=w359:bool)  [unwired: 1 in]
        n224 = case shown="False" w359 {
          tunnel: w358 -> [w368 _]
          tunnel: [w361 w379] -> w357
          tunnel: w356 -> [w360 w379]
          frame False {
            w375 = "Camera"
            w378 = FALSE ("Visible")
            n225 = local read "Camera Settings"() -> (w367:T2)
            n226 = Index Array(array=w368) -> (element=w371:cluster{string[]})  [unwired: 1 in]
            n227 = Unbundle(w367) -> ("Frame Rate"=w366:i32, "Compression"=w365:i32, "Size"=w369:u16)
            n228 = Unbundle(w371) -> (w370:string[])
            n229 = Index Array(array=w370, index=w369) -> (element=w364:string)
            n230 = call-poly <vilib>:"Write Key.vi"("section"=w375, "value"=w364, "key"="Size", "refnum"=w360) -> ("refnum out"=w377:T27)  [unwired: 2 in, 5 out]
            n231 = call-poly <vilib>:"Write Key.vi"("section"=w375, "value"=w366, "key"="FrameRate", "refnum"=w377) -> ("refnum out"=w376:T27)  [unwired: 1 in, 6 out]
            n232 = property on="Camera Settings" class="Clust (strict)"("Visible"=w378) -> ()  [unwired: 2 in, 2 out]
            n233 = local write "DB Camera Config"(w378) -> ()
            n234 = call-poly <vilib>:"Write Key.vi"("section"=w375, "value"=w365, "key"="Compression", "refnum"=w376) -> ("refnum out"=w362:T27)  [unwired: 1 in, 6 out]
            n235 = call <vilib>:"Close Config Data.vi"("refnum"=w362) -> ("file path"=w363:path)  [unwired: 2 in, 8 out]
            n236 = call <vilib>:"Open Config Data.vi"("configuration file path"=w363) -> ("refnum"=w361:T27)  [unwired: 8 in, 2 out]
          }
          frame True {
            n237 = property on="Camera Settings" class="Clust (strict)"("Visible"=TRUE) -> ()  [unwired: 2 in, 2 out]
          }
        }
      }
      event "Camera Settings": Value Change {
        # "Update summary string when any elements of DB camera change"
        n238 = event-data() -> ("NewVal"=w392:T2)  [unwired: 1 in]
        n239 = Index Array(array=w388) -> (element=w387:cluster{string[]})  [unwired: 1 in]
        n240 = Unbundle(w392) -> ("Frame Rate"=w383:i32, "Compression"=w382:i32, "Size"=w385:u16)
        n241 = Unbundle(w387) -> (w386:string[])
        n242 = Index Array(array=w386, index=w385) -> (element=w384:string)
        n243 = Format Into String(format string="%s   %dfps   %d%%", w384, w383, w382) -> (resulting string=w389:string)  [unwired: 2 in, 1 out]
        n244 = Build Array(w389) -> (w390:string[])
        n245 = property on="DB Camera Config" class="Bool (strict)"("Strings [4]"=w390) -> ()  [unwired: 2 in, 2 out]
      }
      event "Motor.Enable": Value Change {
        # "When the test mode otor enable helper is set, update that\ntree row item's value"
        n246 = event-data() -> ("NewVal"=w398:bool)  [unwired: 1 in]
        n247 = Unbundle("Motor") -> ("Value"=w397:dbl)  [unwired: 1 out]
        n248 = Select(t=w397, s=w398, f=0.0) -> (s? t:f=w395:dbl)
        n249 = call <vilib>:"NT Write Number.vi"("Numeric"=w395, "Name"=w394) -> ()  [unwired: 9 in, 1 out]
      }
      event "Test Slider": Value Change {
        # "When the test mode slider helper is set, update that\ntree row item's value"
        n250 = event-data() -> ("NewVal"=w401:dbl)  [unwired: 1 in]
        n251 = call <vilib>:"NT Write Number.vi"("Numeric"=w401, "Name"=w402) -> ()  [unwired: 9 in, 1 out]
      }
      event "On/Off": Value Change {
        # "When the test mode on/off helper value is set, update that\ntree row item's value"
        n252 = event-data() -> ("NewVal"=w406:bool)  [unwired: 1 in]
        n253 = Boolean To (0,1)(Boolean=w406) -> (0, 1=w405:i16)
        n254 = call <vilib>:"NT Write Number.vi"("Numeric"=w405, "Name"=w404) -> ()  [unwired: 9 in, 1 out]
      }
      event "Rev/Fwd": Value Change {
        # "When the test mode helper value for relays is set, update that\ntree row item's value"
        n255 = event-data() -> ("NewVal.Forward"=w414:bool, "NewVal.Reverse"=w413:bool)  [unwired: 1 in]
        n256 = Boolean To (0,1)(Boolean=w414) -> (0, 1=w410:i16)
        n257 = Boolean To (0,1)(Boolean=w413) -> (0, 1=w412:i16)
        n258 = Negate(x=w412) -> (-x=w411:i16)
        n259 = Add(x=w410, y=w411) -> (x+y=w409:i16)
        n260 = call <vilib>:"NT Write Number.vi"("Numeric"=w409, "Name"=w408) -> ()  [unwired: 9 in, 1 out]
      }
      event "Test Ring": Value Change {
        # "When a test mode helper value is selected from the ring,\nset the tree item's variable to the string value"
        n261 = event-data() -> ("NewVal"=w418:u16)  [unwired: 1 in]
        n262 = property on="Test Ring" class="Ring (strict)"() -> ("Strings []"=w419:string[])  [unwired: 2 in, 2 out]
        n263 = Index Array(array=w419, index=w418) -> (element=w417:string)
        n264 = call <vilib>:"NT Write String.vi"("String"=w417, "Name"=w416) -> ()  [unwired: 9 in, 1 out]
      }
      event "Rec Mode": Value Change {
        # "Update globals for recording mode and path to read log from.\nClear when logging and let NetworkTables set path for vision to\nuse."
        n265 = event-data() -> ("NewVal"=w429:enum32{"Stop", "Record", "Playback"})  [unwired: 1 in]
        n266 = global write "WPI_DashboardLogging Global.vi" "Logging Filename"(path "") -> ()
        n267 = case shown="\"Playback\"" w429 {
          tunnel: w428 -> [_ w431 w439]
          tunnel: [_ _ w438] -> w425
          tunnel: [_ _ w437] -> _
          tunnel: w423 -> [_ _ w435]
          tunnel: cluster{i32, i32} {-250, 170} -> [_ _ w434]
          tunnel: [_ _ T30 {"Image Size"=TRUE, "Image Type"=TRUE, "Pixel Value"=TRUE, "ROI Information"=TRUE, "Zoom Factor"=FALSE} ("Image Information Shown:All Elements")] -> w421
          tunnel: [_ _ TRUE ("Zoom Factor")] -> w420
          frame Default {
          }
          frame "Stop", "Record" {
            # "Place Window too"
            n268 = invoke class="VI" method="FP.Close"(reference=w431) -> (reference out=w430:refnum<vi>)  [unwired: 2 in, 2 out]
            n269 = invoke class="VI" method="Abort VI"(reference=w430) -> ()  [unwired: 2 in, 3 out]
          }
          frame "Playback" {
            n270 = call "Open Playback Panel.vi"("Offset"=w434, "DB VI Ref"=w435, "Playback in"=w439) -> ("Playback out"=w436:refnum<vi>)  [unwired: 8 in]
            n271 = register-events(w436) -> (reference out=w438:refnum<event-registration>, error out=w437:errorcluster)  [unwired: 2 in]
          }
        }
        n272 = global write "WPI_DashboardLogging Global.vi" "Recording"(w429) -> ()
        n273 = property on="Camera Image" class="ImageControl"("Image Information Shown"=w421, "Image Information Visible"=w420) -> ()  [unwired: 2 in, 2 out]
        n274 = call <vilib>:"WPI_DashboardNT Log FieldName Cache.vi"("Operation"=enum16{"Lookup/Add", "Index", "Clear"}."Clear") -> ()  [unwired: 8 in, 3 out]
      }
      event Panel Close {
        w440 = enum32{"Stop", "Record", "Playback"}."Stop" ("Rec Mode")
        # "Playback window has been closed, abort"
        n275 = event-data() -> ()  [unwired: 1 in, 4 out]
        n276 = local write "Rec Mode"(w440) -> ()
        n277 = global write "WPI_DashboardLogging Global.vi" "Recording"(w440) -> ()
      }
      event Panel Close {
        # "Abort playback window and ourself"
        n278 = event-data() -> ()  [unwired: 1 in, 4 out]
        n279 = invoke class="VI" method="FP.Close"(reference=w445) -> (reference out=w444:refnum<vi>)  [unwired: 2 in, 2 out]
        n280 = invoke class="VI" method="Abort VI"(reference=w444) -> (error out=w443:errorcluster)  [unwired: 2 in, 2 out]
        n281 = invoke class="VI" method="Abort VI"(error in=w443) -> ()  [unwired: 2 in, 3 out]
      }
      event "Vision": Value Change {
        # "Enable/Disable Compression slider.\nHW USB is hard-coded into the camera"
        n282 = event-data() -> ("NewVal"=w451:u16)  [unwired: 1 in]
        n283 = Equal?(x=w451, y=u32 2 ("milliseconds to wait")) -> (x = y?=w449:bool)
        n284 = Select(t=T31."Disabled and Grayed Out" ("Disabled"), s=w449, f=T31."Enabled" ("Disabled")) -> (s? t:f=w446:T31)
        n285 = property on="Compression" class="Slide (strict)"("DisabledEnum"=w446) -> ()  [unwired: 2 in, 2 out]
      }
    }
  }
  n286 = while {
    tunnel: w38 -> [w454]
    i -> [w457]
    stop <- FALSE stop-if-true
    n287 = Wait (ms)(milliseconds to wait=u32 100) -> ()  [unwired: 1 out]
    n288 = case shown="\"Playback\"" "Rec Mode" {
      tunnel: w457 -> [_ _ w472]
      tunnel: [u32 2829099 ("Base Color") u32 11141120 ("Target Color") w461] -> w453
      frame "Stop", Default {
        # "Reset the color, extra updates don't cost much"
      }
      frame "Record" {
      }
      frame "Playback" {
        # "Playback"
        n289 = Quotient & Remainder(x=w472, y=u32 50 ("milliseconds to wait")) -> (x-y*floor(x/y)=w468:u32)  [unwired: 1 out]
        n290 = Divide(x=w468, y=u32 50 ("milliseconds to wait")) -> (x/y=w465:dbl)
        n291 = Multiply(x=6.283185307179586, y=w465) -> (x*y=w470:dbl)
        n292 = Sine(x=w470) -> (sin(x)=w469:dbl)
        n293 = Absolute Value(x=w469) -> (abs(x)=w462:dbl)
        n294 = call "Interpolate RGB Color.vi"("Proportion"=w462, "Target Color"=u32 30976, "Base Color"=u32 2829099) -> ("Result Color"=w461:u32)  [unwired: 8 in]
      }
    }
    n295 = property class="Pane"(reference=w454, "PaneColor"=w453) -> ()  [unwired: 1 in, 2 out]
  }
  n296 = TCP Create Listener(10:u16 1741 ("timeout ms (25000)")) -> (3:w1:refnum<k5>)  [unwired: 4 in, 2 out]
  n297 = while {
    tunnel: w1 -> [w474]
    stop <- FALSE stop-if-true
    n298 = TCP Wait On Listener(11:w474) -> (4:w473:refnum<k5>)  [unwired: 3 in, 4 out]
    n299 = local write "TCP"(w473) -> ()
  }
  n300 = property on="On/Off" class="Bool (strict)"("Visible"=w6) -> ()  [unwired: 2 in, 2 out]
  n301 = property on="Motor" class="Clust (strict)"("Visible"=w6) -> ()  [unwired: 2 in, 2 out]
  n302 = property on="Progress" class="Clust (strict)"("Visible"=w6) -> ()  [unwired: 2 in, 2 out]
  n303 = property on="Test Ring" class="Ring (strict)"("Visible"=w6) -> ()  [unwired: 2 in, 2 out]
  n304 = property on="Rev/Fwd" class="Clust (strict)"("Visible"=w6) -> ()  [unwired: 2 in, 2 out]
  n305 = property on="Camera Settings" class="Clust (strict)"("Visible"=w6) -> ()  [unwired: 2 in, 2 out]
  n306 = local write "DB Camera Config"(w6) -> ()
  n307 = global write "WPI_DashboardLogging Global.vi" "Recording"(w32) -> ()
  n308 = local write "Rec Mode"(w32) -> ()
